vi "AC & DC Estimator PtByPt.vi"(0 "signal":dbl format="%0.2f", 1 "sample length":i32=100, 2 "initialize":bool) -> (3 "AC estimate (Vrms)":dbl format="%0.2f", 4 "DC estimate (V)":dbl format="%0.2f", 5 "error":i32)   [LabVIEW 2020, in "NI_PtbyPt.lvlib"]
doc: "Computes an estimation of the AC and DC levels of the input <B>signal</B>."
uses:
  NI_PtbyPt.lvlib
  Ramp Pattern by Samples.vi
  NI_AALBase.lvlib
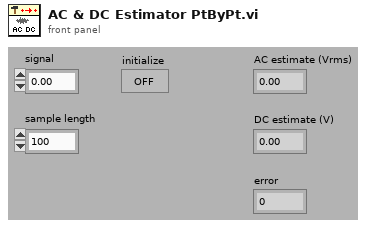
[diagram p1: front panel]
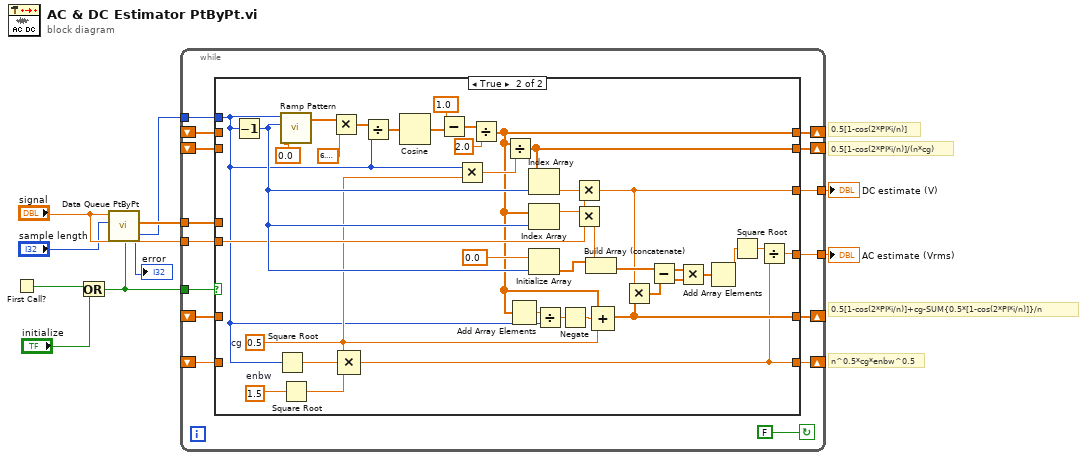
[diagram p0: block diagram]
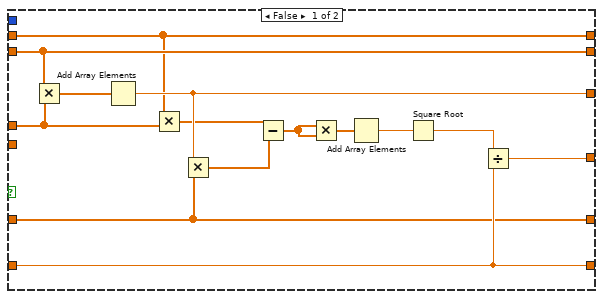
[diagram p2: hidden frame]
diagram:
  # "0.5[1-cos(2*PI*i/n)]"
  # "0.5[1-cos(2*PI*i/n)]+cg-SUM{0.5*[1-cos(2*PI*i/n)]}/n"
  # "n^0.5*cg*enbw^0.5"
  # "0.5[1-cos(2*PI*i/n)]/(n*cg)"
  n1 = First Call?() -> (First Call?: T/F=w3:bool)
  n2 = Or(x=w3, y="initialize") -> (x .or. y?=w2:bool)
  n3 = call "Data Queue PtByPt.vi"("initialize"=w2, "sample length"="sample length", "input data point"="signal") -> ("error"=→"error":i32, "Current Queue"=w7:dbl[], "current length"=w6:i32)  [unwired: 4 in, 2 out]
  n4 = while {
    shift-left: _ -> [w13]
    shift-right: [w14] -> _
    tunnel: [w17] -> w8
    shift-left: _ -> [w15]
    shift-right: [w12] -> _
    shift-left: _ -> [w18]
    shift-right: [w19] -> _
    tunnel: [w20] -> w9
    shift-left: _ -> [w21]
    shift-right: [w22] -> _
    tunnel: w2 -> [w16]
    tunnel: w6 -> [w23]
    tunnel: "signal" -> [w24]
    tunnel: w7 -> [w25]
    stop <- FALSE continue-if-true
    n5 = case shown="True" w16 {
      tunnel: w25 -> [w28 _]
      tunnel: w24 -> [_ w56]
      tunnel: w23 -> [_ w44]
      tunnel: [w32 w66] -> w22
      tunnel: w21 -> [w32 _]
      tunnel: [w38 w49] -> w20
      tunnel: [w34 w41] -> w19
      tunnel: w18 -> [w34 _]
      tunnel: [w33 w40] -> w17
      tunnel: w15 -> [w29 _]
      tunnel: [w27 w52] -> w14
      tunnel: w13 -> [w27 _]
      tunnel: [w29 w45] -> w12
      frame False {
        n6 = Multiply(x=w32, y=w28) -> (x*y=w39:dbl[])
        n7 = Add Array Elements(numeric array=w39) -> (sum=w38:dbl)
        n8 = Multiply(x=w27, y=w28) -> (x*y=w26:dbl[])
        n9 = Multiply(x=w38, y=w29) -> (x*y=w37:dbl[])
        n10 = Subtract(x=w26, y=w37) -> (x-y=w30:dbl[])
        n11 = Multiply(x=w30, y=w30) -> (x*y=w31:dbl[])
        n12 = Add Array Elements(numeric array=w31) -> (sum=w36:dbl)
        n13 = Square Root(x=w36) -> (sqrt(x)=w35:dbl)
        n14 = Divide(x=w35, y=w34) -> (x/y=w33:dbl)
      }
      frame True {
        w50 = 0.5  # cg
        w64 = 1.5  # enbw
        n15 = Decrement(x=w44) -> (x-1=w58:i32)
        n16 = Square Root(x=w44) -> (sqrt(x)=w62:dbl)
        n17 = call-poly "Ramp Pattern.vi"("start"=0.0, "end"=w58, "samples"=w44) -> ("Ramp Pattern"=w75:dbl[])  [unwired: 7 in, 1 out]
        n18 = Square Root(x=w64) -> (sqrt(x)=w63:dbl)
        n19 = Multiply(x=w75, y=6.283185307179586) -> (x*y=w73:dbl[])
        n20 = Compound Arithmetic op=MULTIPLY(w50, w62, w63) -> (w41:dbl)
        n21 = Divide(x=w73, y=w44) -> (x/y=w71:dbl[])
        n22 = Cosine(x=w71) -> (cos(x)=w70:dbl[])
        n23 = Subtract(x=1.0, y=w70) -> (x-y=w69:dbl[])
        n24 = Multiply(x=w44, y=w50) -> (x*y=w67:dbl)
        n25 = Divide(x=w69, y=2.0) -> (x/y=w52:dbl[])
        n26 = Divide(x=w52, y=w67) -> (x/y=w66:dbl[])
        n27 = Add Array Elements(numeric array=w52) -> (sum=w54:dbl)
        n28 = Index Array(array=w66, index=w58) -> (element=w65:dbl)
        n29 = Index Array(array=w52, index=w58) -> (element=w57:dbl)
        n30 = Initialize Array(0.0 ("Element Data"), w58) -> (w60:dbl[])
        n31 = Divide(x=w54, y=w44) -> (x/y=w53:dbl)
        n32 = Negate(x=w53) -> (-x=w51:dbl)
        n33 = Multiply(x=w65, y=w56) -> (x*y=w49:dbl)
        n34 = Multiply(x=w57, y=w56) -> (x*y=w55:dbl)
        n35 = Build Array (concatenate)(w60, w55) -> (w59:dbl[])
        n36 = Compound Arithmetic op=ADD(w52, w51, w50) -> (w45:dbl[])
        n37 = Multiply(x=w49, y=w45) -> (x*y=w48:dbl[])
        n38 = Subtract(x=w59, y=w48) -> (x-y=w47:dbl[])
        n39 = Multiply(x=w47, y=w47) -> (x*y=w46:dbl[])
        n40 = Add Array Elements(numeric array=w46) -> (sum=w43:dbl)
        n41 = Square Root(x=w43) -> (sqrt(x)=w42:dbl)
        n42 = Divide(x=w42, y=w41) -> (x/y=w40:dbl)
      }
    }
  }
  "DC estimate (V)" <- w9
  "AC estimate (Vrms)" <- w8
